vi "ad get next run.vi"(7 "p":u32[](array[numeric]), 8 "error in (no error)":errorcluster, 9 "run":u32, 10 "state":T1, 11 "adh":i32) -> (0 "error out":errorcluster, 1 "run out":u32, 2 "state out":T1, 3 "function return":i32, 5 "p out":u32[](array[numeric]))   [LabVIEW 2021, in "libad4.lvlib"]
doc: "LIBAD4 function: ad_get_next_run (int32_t adh, struct ad_scan_state *state, uint32_t *run, void *p);\n\nReturns the measurements from a scan run. Returns measurements directly from the DAQ (does not convert them from binary representation to float). Bytes are returned in \"network byte order\", not x86 order."
uses:
  <userlib>/libad4/libad4.lvlib
  <userlib>/libad4/controls/ad scan state.ctl
  <userlib>/libad4/libad4.dll
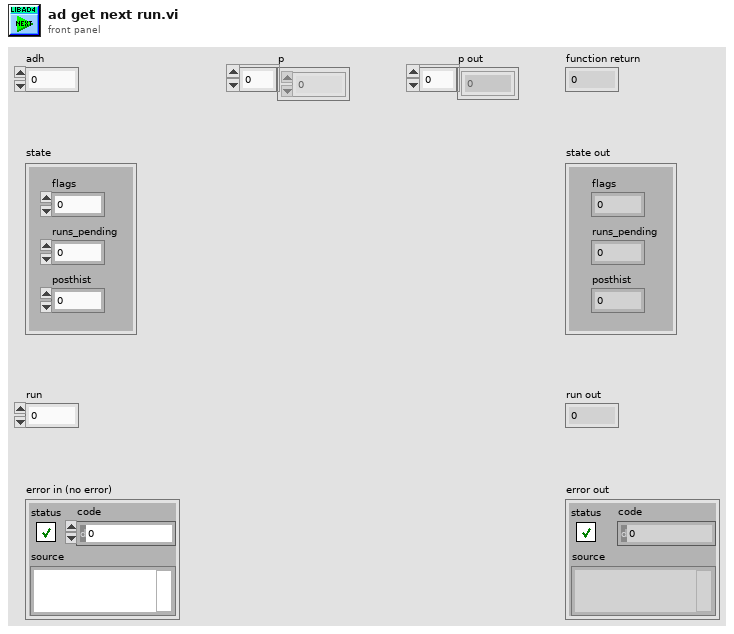
[diagram p1: front panel]
types:
  T1 = typedef "libad4.lvlib/ad scan state.ctl" = cluster{"flags":i32, "runs_pending":i32, "posthist":i64}
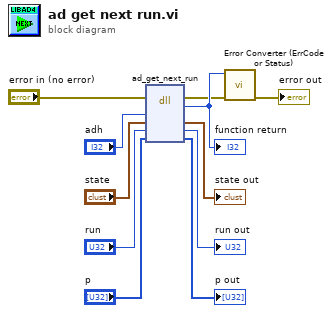
[diagram p0: block diagram]
diagram:
  n1 = dll-call lib="C:/Program Files/National Instruments/LabVIEW 2021/user.lib/libad4/libad4.*" fn="ad_get_next_run"(error in="error in (no error)", "adh"="adh", "state"="state", "run"="run", "p"="p") -> (error out=w2:errorcluster, "return type"=w11:i32, "state"=→"state out":T1, "run"=→"run out":u32, "p"=→"p out":u32[])  [unwired: 3 in, 1 out]
  "function return" <- w11
  n2 = call <userlib>:"Error Converter (ErrCode or Status).vi"("error in (no error)"=w2, "error code"=w11) -> ("error out"=→"error out":errorcluster)  [unwired: 9 in]
